vi "DoorAccess-.vi"() -> ()   [LabVIEW 2011]
uses:
  <vilib>/Platform/TimedLoop/XDataNode/timing_clust.ctl
  <vilib>/Platform/TimedLoop/XDataNode/nitl_modes.ctl
  <vilib>/Platform/TimedLoop/XDataNode/wakeup.ctl
  Variable/gSTOP.vi
  Routine/Queue/Alert.vi
  Routine/Queue/Card.vi
  Routine/DoorTread/Alerts.vi
  Routine/DoorTread/Tread_03.vi
  Routine/DoorTread/Tread_01.vi
  Routine/DoorTread/Tread_02.vi
  <vilib>/Platform/TimedLoop/XDataNode/XDataNode.xnode
  <vilib>/Platform/TimedLoop/XDataNode/XDNodeRunTimeDep.lvlib
panel:
  in  "Stop":bool
  out "Certificate":bool
  in  "En3":bool
  in  "ID 3":u8=3
  in  "IP 3":string="192.168.1.128"
  in  "Port 3":u16=1621
  in  "Node 3":u8=3
  in  "ID 1":u8=1
  in  "IP 1":string="192.168.1.126"
  in  "Port 1":u16=1621
  in  "Node 1":u8=1
  in  "Node 2":u8=3
  in  "Port 2":u16=1621
  in  "IP 2":string="192.168.1.127"
  in  "ID 2":u8=2
  in  "En2":bool
  out "Card Info":string="002001/22548:59693"
  in  "En1":bool
  in  "En0":bool
  in  "ID 0":u8
  in  "IP 0":string="10.156.16.65"
  in  "Port 0":u16=6341
  # "Door Access System v0.1\nDesigner : Ares.Chung"
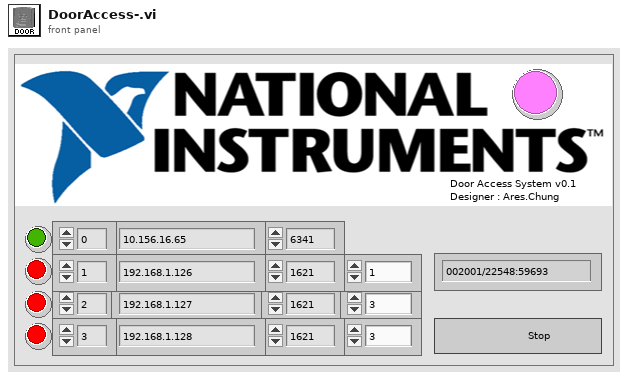
[diagram p1: front panel]
types:
  T1 = enum16{"Obtain", "Enqueue", "Dequeue", "Release"}
  T2 = typedef "XDNodeRunTimeDep.lvlib/timing_clust.ctl" = cluster{"Expected End [f-1]":u64, "Actual End [f-1]":u64, "Finished Late? [f-1]":bool, "Expected End [i-1]":u64, "Actual End [i-1]":u64, "Finished Late? [i-1]":bool, "Expected Start [i]":u64, "Actual Start [i]":u64, "Expected Start [f]":u64, "Actual Start [f]":u64, "Source Name":string, "Structure Name":string, "Period":i64, "Deadline":i64, "Offset":i64, "Start":i64, "Priority":i32, "Timeout":i32, "Mode":T3, "Wakeup Reason":T4, "Error":errorcluster, "Source Type":string, "Secondary Source Type":string, "Global End Time":u64, "Global Start Time":u64, "Frame Duration":u64, "Iteration Duration":u64, "Assigned CPU":i32, "I/O Scan Engine Mode":u32}
  T3 = typedef "XDNodeRunTimeDep.lvlib/nitl_modes.ctl" = enum32{"No Change", "Process missed periods, maintain original phase", "Discard missed periods, maintain original phase", "Process missed periods, ignore original phase", "Discard missed periods, ignore original phase"}
  T4 = typedef "XDNodeRunTimeDep.lvlib/wakeup.ctl" = enum32{"Normal", "Aborted", "Asynchronous wakeup", "Timing source error", "Timed loop error", "Timeout"}
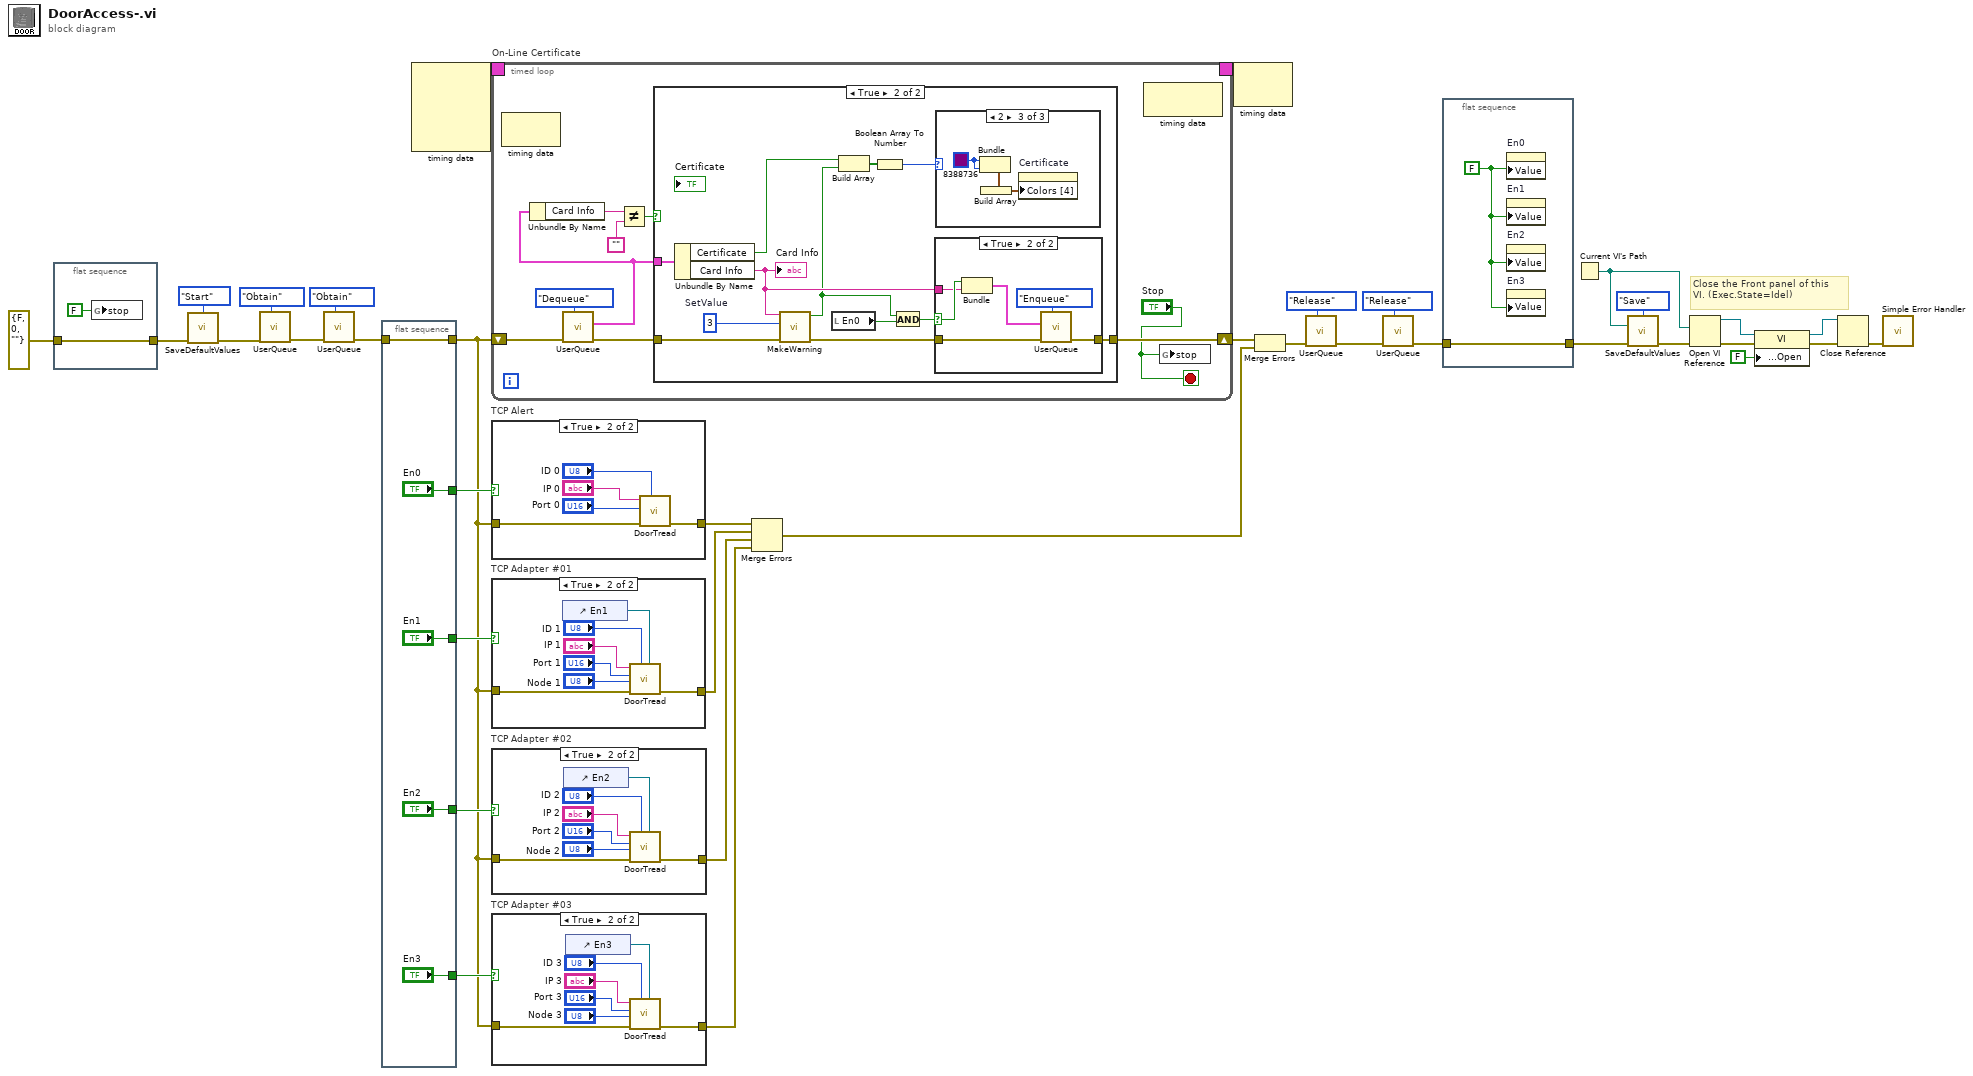
[diagram p0: block diagram]
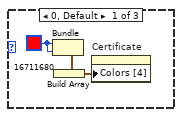
[diagram p4: hidden frame]
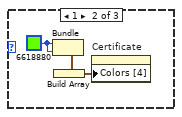
[diagram p5: hidden frame]
diagram:
  # "Close the Front panel of this\nVI. (Exec.State=Idel)"
  n1 = flat-sequence {
    tunnel: errorcluster {"status"=FALSE, "code"=0, "source"=""} ("error constant") -> [w37]
    tunnel: [w37] -> w14
    frame #0 {
      n2 = global write "gSTOP.vi" "stop"(FALSE ("stop")) -> ()
    }
  }
  n3 = call "SaveDefaultValues.vi"("Step"=enum16{"Start", "Save"}."Start", "error in (no error)"=w14) -> ("error out"=w13:errorcluster)  [unwired: 13 in]
  n4 = call-poly "UserQueue.vi"("Mode"=T1."Obtain", "error in (no error)"=w13) -> ("error out"=w21:errorcluster)  [unwired: 8 in, 1 out]
  n5 = call-poly "UserQueue.vi"("Mode"=T1."Obtain", "error in (no error)"=w21) -> ("error out"=w16:errorcluster)  [unwired: 8 in, 1 out]
  n6 = flat-sequence {
    tunnel: ["En2"] -> w34
    tunnel: ["En1"] -> w33
    tunnel: ["En3"] -> w24
    tunnel: ["En0"] -> w18
    tunnel: w16 -> [w39]
    tunnel: [w39] -> w15
    frame #0 {
    }
  }
  n7 = node-c288() -> (w27:T2)  [unwired: 4 in]
  n8 = timed-loop "On-Line Certificate" {
    shift-right: [w47] -> w29
    shift-left: w15 -> [w51]
    timing: w27 -> [_]
    timing-out: [_] -> w26
    stop <- "Stop" stop-if-true
    n9 = node-c288() -> ()  [unwired: 1 in, 1 out]
    n10 = call-poly "UserQueue.vi"("Mode"=T1."Dequeue", "error in (no error)"=w51) -> ("error out"=w48:errorcluster, "Queue Out"=w46:cluster{"Certificate":bool, "Card Info":string})  [unwired: 8 in]
    n11 = Unbundle By Name(w46) -> ("Card Info"=w50:string)
    n12 = Not Equal?(x=w50, y="") -> (x != y?=w49:bool)
    n13 = case shown="True" w49 {
      tunnel: w48 -> [w55 w66]
      tunnel: [w55 w64] -> w47
      tunnel: w46 -> [_ w67]
      frame False {
      }
      frame True {
        w62 = u8 3  # SetValue
        n14 = Unbundle By Name(w67) -> ("Certificate"=w59:bool, "Card Info"=w63:string)
        "Card Info" <- w63
        n15 = call "MakeWarning.vi"("error in (no error)"=w66, "Setup"=w62, "String"=w63) -> ("error out"=w65:errorcluster, "Warning"=w58:bool)  [unwired: 7 in]
        n16 = local read "En0"() -> (w61:bool)
        n17 = Build Array(w59, w58) -> (w57:bool[])
        n18 = Boolean Array To Number(Boolean array=w57) -> (number=w56:u32)
        n19 = And(x=w58, y=w61) -> (x .and. y?=w60:bool)
        n20 = case shown="True" w60 {
          selector: w60 -> [_ w80]
          tunnel: w65 -> [w77 w82]
          tunnel: [w77 w81] -> w64
          tunnel: w63 -> [_ w79]
          frame False {
          }
          frame True {
            n21 = Bundle(w80, "Card Info"=w79) -> (w78:cluster{bool, "Card Info":string})  [unwired: 1 in]
            n22 = call-poly "UserQueue.vi"("Mode"=T1."Enqueue", "error in (no error)"=w82, "Queue In"=w78) -> ("error out"=w81:errorcluster)  [unwired: 7 in, 1 out]
          }
        }
        n23 = case shown="2" w56 {
          frame 0, Default {
            w70 = u32 16711680 ("Color Box")
            n24 = Bundle("Color Box"=w70, "Color Box"=w70) -> (w69:cluster{"Color Box":u32, "Color Box":u32})  [unwired: 1 in]
            n25 = Build Array(w69) -> (w68:cluster{"Color Box":u32, "Color Box":u32}[])
            n26 = property on="Certificate" class="Bool (strict)"("Colors [4]"=w68) -> ()  [unwired: 2 in, 2 out]
          }
          frame 1 {
            w73 = u32 6618880 ("Color Box")
            n27 = Bundle("Color Box"=w73, "Color Box"=w73) -> (w72:cluster{"Color Box":u32, "Color Box":u32})  [unwired: 1 in]
            n28 = Build Array(w72) -> (w71:cluster{"Color Box":u32, "Color Box":u32}[])
            n29 = property on="Certificate" class="Bool (strict)"("Colors [4]"=w71) -> ()  [unwired: 2 in, 2 out]
          }
          frame 2 {
            w76 = u32 8388736 ("Color Box")
            n30 = Bundle("Color Box"=w76, "Color Box"=w76) -> (w75:cluster{"Color Box":u32, "Color Box":u32})  [unwired: 1 in]
            n31 = Build Array(w75) -> (w74:cluster{"Color Box":u32, "Color Box":u32}[])
            n32 = property on="Certificate" class="Bool (strict)"("Colors [4]"=w74) -> ()  [unwired: 2 in, 2 out]
          }
        }
      }
    }
    n33 = node-c288() -> ()  [unwired: 1 in, 1 out]
    n34 = global write "gSTOP.vi" "stop"("Stop") -> ()
  }
  n35 = case "TCP Alert" shown="True" w18 {
    tunnel: w15 -> [w84 w89]
    tunnel: [w84 w85] -> w25
    frame False {
    }
    frame True {
      n36 = call-poly "DoorTread.vi"("ID"="ID 0", "error in (no error)"=w89, "Port"="Port 0", "IP"="IP 0") -> ("error out"=w85:errorcluster)  [unwired: 7 in]
    }
  }
  n37 = case "TCP Adapter #01" shown="True" w33 {
    tunnel: w15 -> [w90 w97]
    tunnel: [w90 w93] -> w31
    frame False {
    }
    frame True {
      n38 = control-ref of="En1"() -> (w91:refnum<vi>)
      n39 = call-poly "DoorTread.vi"("Bool Refnum"=w91, "ID"="ID 1", "error in (no error)"=w97, "Number"="Node 1", "Port"="Port 1", "IP"="IP 1") -> ("error out"=w93:errorcluster)  [unwired: 5 in]
    }
  }
  n40 = case "TCP Adapter #02" shown="True" w34 {
    tunnel: w15 -> [w98 w105]
    tunnel: [w98 w100] -> w30
    frame False {
    }
    frame True {
      n41 = control-ref of="En2"() -> (w99:refnum<vi>)
      n42 = call-poly "DoorTread.vi"("Bool Refnum"=w99, "ID"="ID 2", "error in (no error)"=w105, "Number"="Node 2", "Port"="Port 2", "IP"="IP 2") -> ("error out"=w100:errorcluster)  [unwired: 5 in]
    }
  }
  n43 = case "TCP Adapter #03" shown="True" w24 {
    tunnel: w15 -> [w106 w113]
    tunnel: [w106 w108] -> w23
    frame False {
    }
    frame True {
      n44 = control-ref of="En3"() -> (w107:refnum<vi>)
      n45 = call-poly "DoorTread.vi"("Bool Refnum"=w107, "ID"="ID 3", "error in (no error)"=w113, "Number"="Node 3", "Port"="Port 3", "IP"="IP 3") -> ("error out"=w108:errorcluster)  [unwired: 5 in]
    }
  }
  n46 = Merge Errors(w25, w31, w30, w23) -> (w28:errorcluster)
  n47 = node-c288(w26) -> ()  [unwired: 1 out]
  n48 = Merge Errors(w29, w28) -> (w32:errorcluster)
  n49 = call-poly "UserQueue.vi"("Mode"=T1."Release", "error in (no error)"=w32) -> ("error out"=w19:errorcluster)  [unwired: 8 in, 1 out]
  n50 = call-poly "UserQueue.vi"("Mode"=T1."Release", "error in (no error)"=w19) -> ("error out"=w2:errorcluster)  [unwired: 8 in, 1 out]
  n51 = flat-sequence {
    tunnel: w2 -> [w115]
    tunnel: [w115] -> w1
    frame #0 {
      w114 = FALSE
      n52 = property on="En0" class="Bool (strict)"("Value"=w114) -> ()  [unwired: 2 in, 2 out]
      n53 = property on="En1" class="Bool (strict)"("Value"=w114) -> ()  [unwired: 2 in, 2 out]
      n54 = property on="En2" class="Bool (strict)"("Value"=w114) -> ()  [unwired: 2 in, 2 out]
      n55 = property on="En3" class="Bool (strict)"("Value"=w114) -> ()  [unwired: 2 in, 2 out]
    }
  }
  n56 = Current VI's Path() -> (path=w3:path)
  n57 = call "SaveDefaultValues.vi"("Step"=enum16{"Start", "Save"}."Save", "VI to save"=w3, "error in (no error)"=w1) -> ("error out"=w5:errorcluster)  [unwired: 12 in]
  n58 = Open VI Reference(vi path=w3, error in (no error)=w5) -> (vi reference=w10:refnum<vi>, error out=w9:errorcluster)  [unwired: 4 in]
  n59 = property class="VI"(reference=w10, error in=w9, "Front Panel Window:Open"=FALSE) -> (reference out=w8:refnum<vi>, error out=w6:errorcluster)
  n60 = Close Reference(reference=w8, error in (no error)=w6) -> (error out=w4:errorcluster)
  n61 = call <vilib>:"Simple Error Handler.vi"("error in (no error)"=w4) -> ()  [unwired: 4 in, 5 out]
